vi "GetDataUnits.vi"(8 "error in (no error)":errorcluster caption="entrée d'erreur (pas d'erreur)", 11 "Device en entrée":refnum<class "BaseDevice.lvclass">) -> (0 "error out":errorcluster caption="sortie d'erreur", 2 "DataUnits":string[][](array[string]), 3 "Device en sortie":refnum<class "BaseDevice.lvclass">)   [LabVIEW 2019, in "BaseDevice.lvclass"]
uses:
  BaseDevice.lvclass
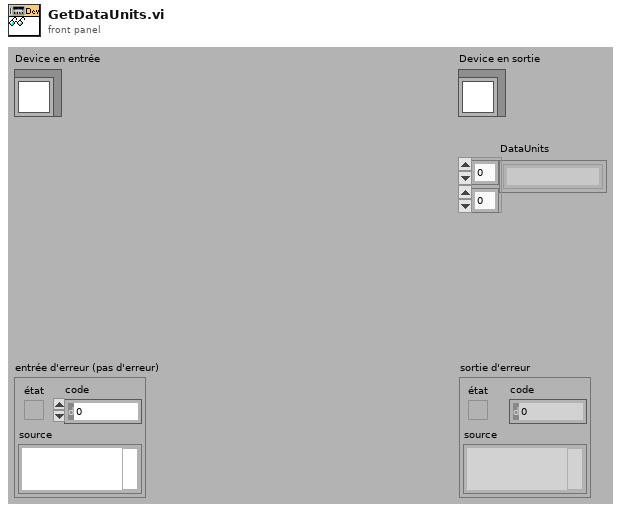
[diagram p1: front panel]
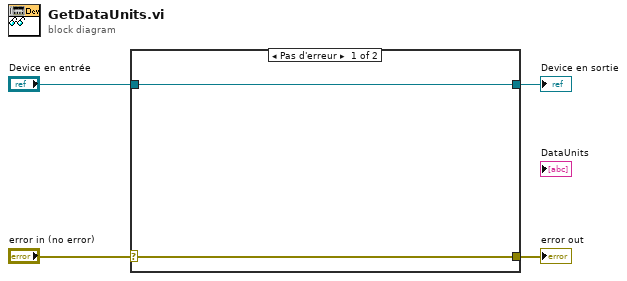
[diagram p0: block diagram]
diagram:
  n1 = case shown="Pas d'erreur" "error in (no error)" {
    selector: "error in (no error)" -> [w6 w7]
    tunnel: [w6 w7] -> w3
    tunnel: [w5 w8] -> w1
    tunnel: "Device en entrée" -> [w5 w8]
    frame No Error {
    }
    frame Error {
    }
  }
  "error out" <- w3
  "Device en sortie" <- w1
